vi "generateWaveform.vi"(8 "error in (no error)":errorcluster, 11 "SquareWave in":refnum<class "SquareWave.lvclass">) -> (0 "error out":errorcluster, 2 "Output":dbl, 3 "SquareWave out":refnum<class "SquareWave.lvclass">)   [LabVIEW 2015, in "SquareWave.lvclass"]
uses:
  SquareWave.lvclass
  <vilib>/ptbypt/NI_PtbyPt.lvlib
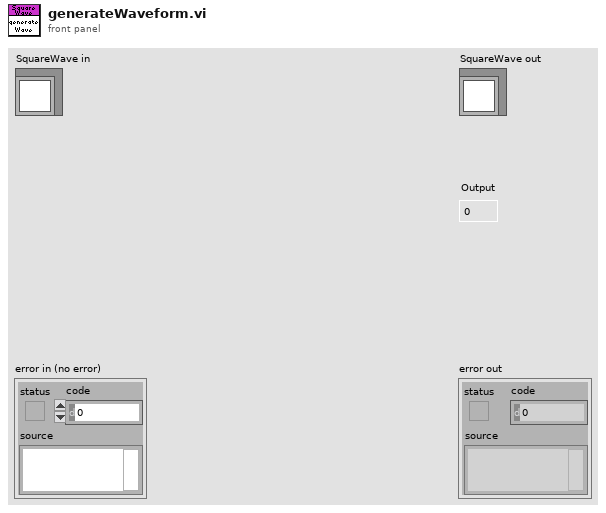
[diagram p1: front panel]
types:
  T1 = typedef "FAMTTypedefs.lvlib/DutyCycle.ctl" = dbl
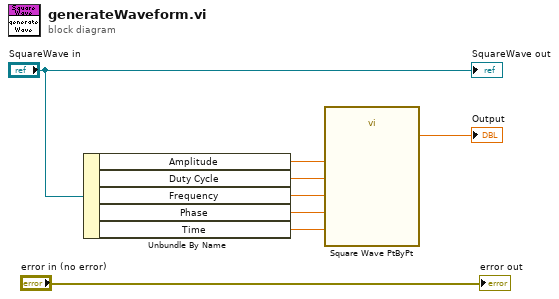
[diagram p0: block diagram]
diagram:
  n1 = Unbundle By Name("SquareWave in") -> ("Amplitude"=w7:dbl, "Duty Cycle"=w6:T1, "Frequency"=w5:dbl, "Phase"=w4:dbl, "Time"=w3:dbl)
  n2 = call <vilib>:"Square Wave PtByPt.vi"("amplitude"=w7, "frequency"=w5, "phase"=w4, "time"=w3, "duty cycle (%)"=w6) -> ("square wave"=→"Output":dbl)
  "error out" <- "error in (no error)"
  "SquareWave out" <- "SquareWave in"
